vi "Pkt - Menu Data Types.vi"() -> (2 "Menu Tags":string[](array[string])=["CTBoolean", "CTSingle", "CTDouble", "CTI8", "CTI16", "CTI32", "CTI64", "CTU8", "CTU16", "CTU32", "CTU64"], 3 "Menu Names":string[](array[string])=["Boolean", "Single", "Double", "I8", "I16", "I32", "I64", "U8", "U16", "U32", "U64"])   [LabVIEW 2016, in "UDP-Custom-Device System Explorer.lvlib"]
uses:
  UDP-Custom-Device System Explorer.lvlib
  Shared/Types/Shared - Channel Data Type.ctl
  Shared/UDP-Custom-Device Shared.lvlib
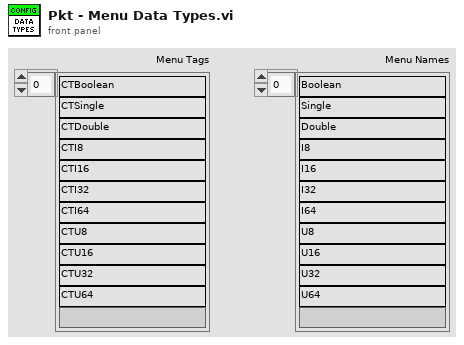
[diagram p1: front panel]
types:
  T1 = typedef "UDP-Custom-Device Shared.lvlib/Shared - Channel Data Type.ctl" = enum16{"Boolean", "Single", "Double", "I8", "I16", "I32", "I64", "U8", "U16", "U32", "U64"}
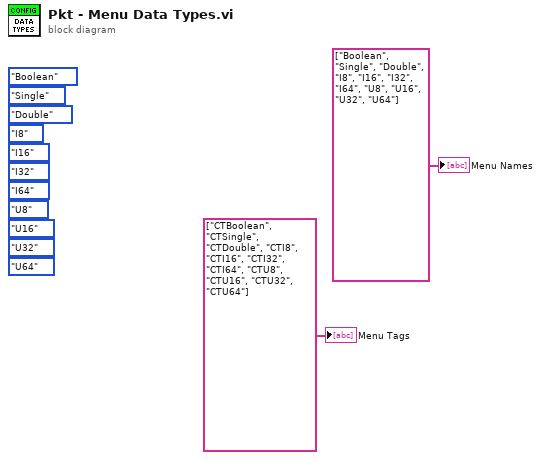
[diagram p0: block diagram]
diagram:
  (unwired) Shared_-_Channel_Data_Type."U64" ("Data Type")
  (unwired) Shared_-_Channel_Data_Type."U32" ("Data Type")
  (unwired) Shared_-_Channel_Data_Type."U16" ("Data Type")
  (unwired) Shared_-_Channel_Data_Type."U8" ("Data Type")
  (unwired) Shared_-_Channel_Data_Type."I64" ("Data Type")
  (unwired) Shared_-_Channel_Data_Type."I32" ("Data Type")
  (unwired) Shared_-_Channel_Data_Type."I16" ("Data Type")
  (unwired) Shared_-_Channel_Data_Type."I8" ("Data Type")
  (unwired) Shared_-_Channel_Data_Type."Double" ("Data Type")
  (unwired) Shared_-_Channel_Data_Type."Single" ("Data Type")
  (unwired) Shared_-_Channel_Data_Type."Boolean" ("Data Type")
  "Menu Names" <- string[] ["Boolean", "Single", "Double", "I8", "I16", "I32", "I64", "U8", "U16", "U32", "U64"] ("item names")
  "Menu Tags" <- string[] ["CTBoolean", "CTSingle", "CTDouble", "CTI8", "CTI16", "CTI32", "CTI64", "CTU8", "CTU16", "CTU32", "CTU64"] ("item names")
